vi "Clear Transformation.vi"(8 "error in (no error)":errorcluster, 11 "Object Refnum In":refnum<vi>) -> (0 "error out":errorcluster, 3 "Object Refnum Out":refnum<vi>)   [LabVIEW 2020, in "NI_3D Picture Control.lvlib"]
doc: "Clears any transformations previously applied to an object in a 3D scene by modifying the identity matrices that describe the transformations."
uses:
  <vilib>/picture/3D Picture Control/NI_3D Picture Control.lvlib
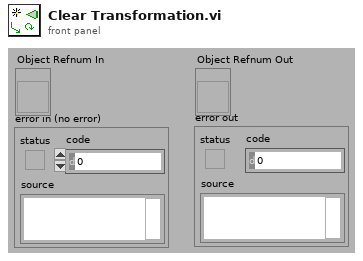
[diagram p1: front panel]
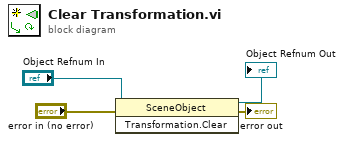
[diagram p0: block diagram]
diagram:
  n1 = invoke class="SceneObject" method="Transformation.Clear"(reference="Object Refnum In", error in="error in (no error)") -> (reference out=→"Object Refnum Out":refnum<vi>, error out=→"error out":errorcluster)  [unwired: 1 in, 1 out]
